vi "Knob1.vi"(0 "Freqin":dbl=1000.0 format="%_7g", 2 "Knob":i8(knob)=1 scale=1.0..20.0, 3 "Frequency Step Size":i32(ring)=7 items=["0.1Hz", "1Hz", "10Hz", "100Hz", "1KHz", "10KHz", "100KHz", "1MHz", "10MHz", "100MHz", "1GHz"], 4 "Reset":bool, 5 "fup":bool, 6 "fdn":bool) -> (8 "freqcommand":string, 10 "freqout":dbl)   [LabVIEW 2017]
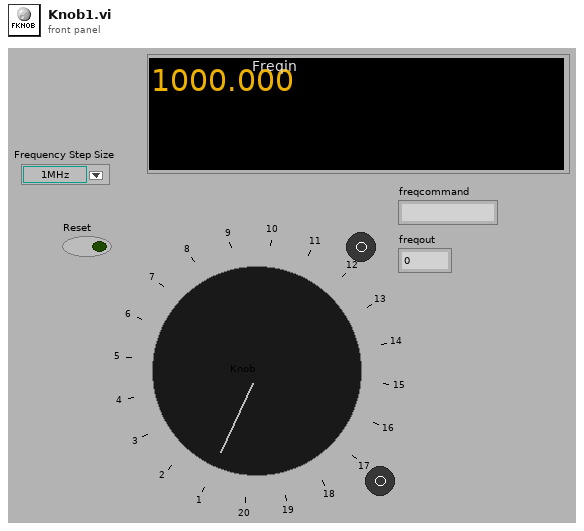
[diagram p1: front panel]
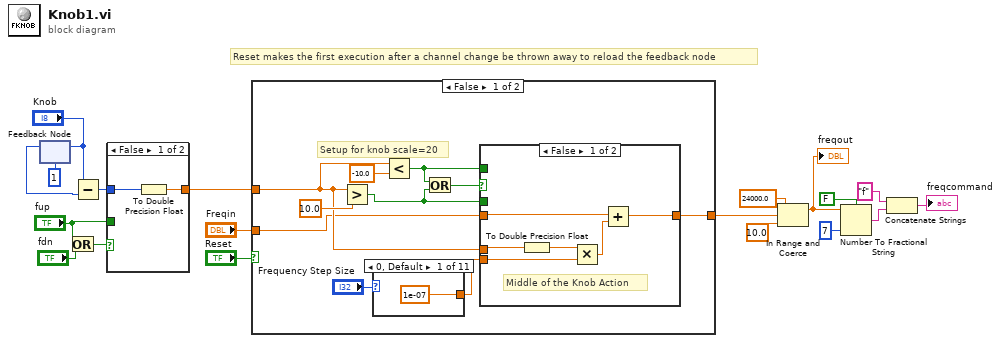
[diagram p0: block diagram]
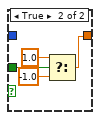
[diagram p2: hidden frame]
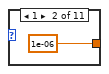
[diagram p3: hidden frame]
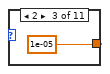
[diagram p4: hidden frame]
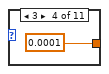
[diagram p5: hidden frame]
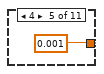
[diagram p6: hidden frame]
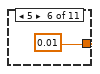
[diagram p7: hidden frame]
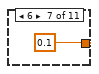
[diagram p8: hidden frame]
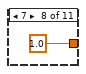
[diagram p9: hidden frame]
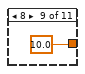
[diagram p10: hidden frame]
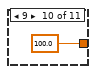
[diagram p11: hidden frame]
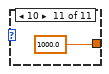
[diagram p12: hidden frame]
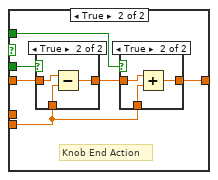
[diagram p13: hidden frame]
diagram:
  # "Reset makes the first execution after a channel change be thrown away to reload the feedback node"
  n1 = feedback-in #1("Knob") -> ()
  n2 = feedback #1(i8 1 ("Knob")) -> (w18:i8)
  n3 = Or(x="fup", y="fdn") -> (x .or. y?=w5:bool)
  n4 = Subtract(x="Knob", y=w18) -> (x-y=w3:i8)
  n5 = case shown="False" w5 {
    tunnel: w3 -> [w20 _]
    tunnel: [w21 w24] -> w2
    tunnel: "fup" -> [_ w25]
    frame False {
      n6 = To Double Precision Float(number=w20) -> (double precision float=w21:dbl)
    }
    frame True {
      n7 = Select(t=1.0, s=w25, f=-1.0) -> (s? t:f=w24:dbl)
    }
  }
  n8 = case shown="False" "Reset" {
    tunnel: w2 -> [w30 _]
    tunnel: "Freqin" -> [w29 w67]
    tunnel: [w28 w67] -> w12
    frame False {
      # "Setup for knob scale=20"
      n9 = Greater?(x=w30, y=10.0) -> (0:w32:bool)
      n10 = case shown="0, Default" "Frequency Step Size" {
        tunnel: [1e-07 1e-06 1e-05 0.0001 0.001 0.01 0.1 1.0 10.0 100.0 1000.0] -> w27
        frame 0, Default {
        }
        frame 1 {
        }
        frame 2 {
        }
        frame 3 {
        }
        frame 4 {
        }
        frame 5 {
        }
        frame 6 {
        }
        frame 7 {
        }
        frame 8 {
        }
        frame 9 {
        }
        frame 10 {
        }
      }
      n11 = Less?(x=w30, y=-10.0) -> (x < y?=w31:bool)
      n12 = Or(x=w31, y=w32) -> (x .or. y?=w33:bool)
      n13 = case shown="False" w33 {
        tunnel: w32 -> [_ w58]
        tunnel: w29 -> [w51 w57]
        tunnel: w31 -> [_ w55]
        tunnel: [w52 w54] -> w28
        tunnel: w27 -> [w50 w53]
        tunnel: w30 -> [w47 _]
        frame False {
          # "Middle of the Knob Action"
          n14 = To Double Precision Float(number=w47) -> (double precision float=w48:dbl)
          n15 = Multiply(x=w48, y=w50) -> (x*y=w49:dbl)
          n16 = Add(x=w51, y=w49) -> (x+y=w52:dbl)
        }
        frame True {
          # "Knob End Action"
          n17 = case shown="True" w58 {
            tunnel: w57 -> [w63 w65]
            tunnel: [w63 w66] -> w56
            tunnel: w53 -> [_ w64]
            frame False {
            }
            frame True {
              n18 = Subtract(x=w65, y=w64) -> (x-y=w66:dbl)
            }
          }
          n19 = case shown="True" w55 {
            tunnel: w56 -> [w59 w61]
            tunnel: [w59 w62] -> w54
            tunnel: w53 -> [_ w60]
            frame False {
            }
            frame True {
              n20 = Add(x=w61, y=w60) -> (x+y=w62:dbl)
            }
          }
        }
      }
    }
    frame True {
    }
  }
  n21 = In Range and Coerce(upper limit=24000.0, x=w12, lower limit=10.0) -> (coerced(x)=w9:dbl)  [unwired: 1 out]
  "freqout" <- w9
  n22 = Number To Fractional String(use system decimal point (T)=FALSE, number=w9, precision (6)=i16 7) -> (F-format string=w8:string)  [unwired: 1 in]
  n23 = Concatenate Strings("f" ("element"), w8) -> (→"freqcommand":string)
